vi "数组的更多使用3.vi"() -> ()   [LabVIEW 2025]
uses:
  87c27d12-5d39-4814-956f-28ff39b3eca0.vi
  7a71da50-a804-472e-9fb4-ea32467be636.vi
  161af4c8-741e-4c3b-a09d-9f8106a9c38e.vi
  <vilib>/Array/Sort 2D Array - Pop Stack.vi
  <vilib>/Array/Sort 2D Array - Push Stack.vi
  7a71da50-a804-472e-9fb4-ea32467be636.vi/269d4b3b-47f5-49e3-8884-44851e4dd9d5.vi
  7a71da50-a804-472e-9fb4-ea32467be636.vi/6d99389c-673d-4efb-bf33-19b32bcf4cf8.vi
panel:
  out "数组 4":cluster{"数值":dbl, "字符串":string}[](array[cluster])
  in  "数组 3":T1(array[cluster])
  out "簇 3":cluster{"数值":dbl, "字符串":string}
  out "数值 2":dbl
  out "字符串":string
  out "数值":dbl
  out "布尔":bool
  in  "簇 2":T2
  in  "数组":T1(array[cluster])
  out "簇":T2
  out "转置的数组":dbl[][](array[numeric])
  out "shuffled array 2":dbl[][](array[numeric]) caption="重排后数组"
  out "sorted 2D array":dbl[][](array[numeric]) caption="排序后的二维数组"
  out "index out of range?":bool caption="索引超出范围？"
  in  "dimension to index (column)":enum16{"column", "row"}(ring) caption="要索引的维度（列）"
  in  "index":i32 caption="索引"
  in  "二维数组":dbl[][](array[numeric])
  out "y值":dbl
  in  "分数索引":dbl
  out "降采样的数组 2":dbl[](array[numeric])
  out "降采样的数组 1":dbl[](array[numeric])
  in  "数组 2":dbl[](array[numeric])
  out "交织的数组":dbl[](array[numeric])
  in  "第n个元素":dbl
  out "数组（最后n个元素置于前端）":dbl[](array[numeric])
  out "shuffled array":dbl[](array[numeric]) caption="重排一维数组"
  out "1维数组排序":dbl[](array[numeric])
  in  "数组 1":dbl[](array[numeric])
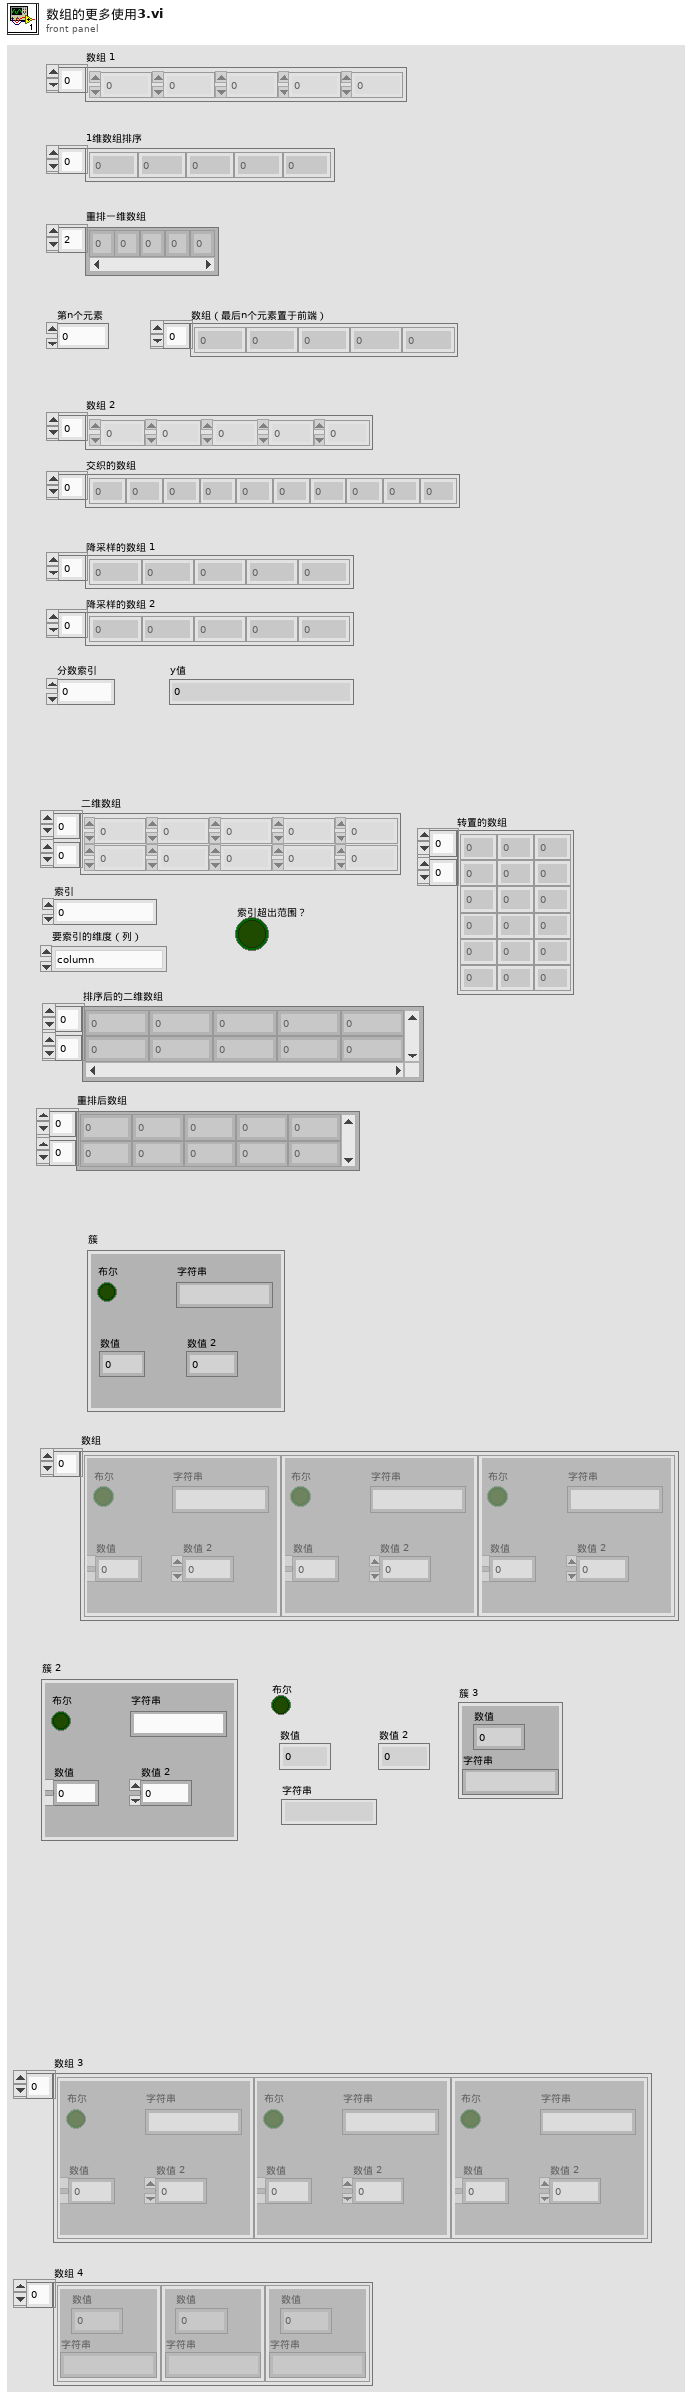
[diagram p1: front panel]
types:
  T1 = cluster{"布尔":bool, "数值":dbl, "字符串":string, "数值 2":dbl}[]
  T2 = cluster{"布尔":bool, "数值":dbl, "字符串":string, "数值 2":dbl}
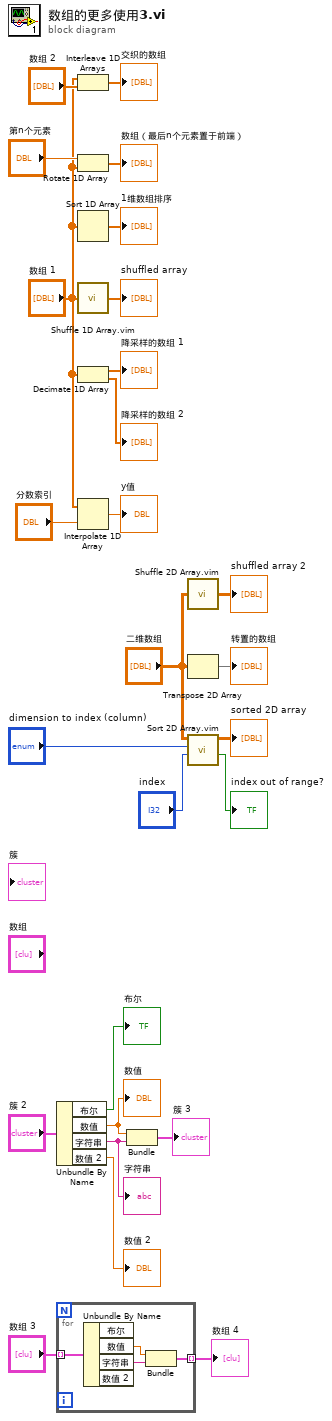
[diagram p0: block diagram]
diagram:
  n1 = Unbundle By Name("簇 2") -> ("布尔"=→"布尔":bool, "数值"=w5:dbl, "字符串"=w4:string, "数值 2"=→"数值 2":dbl)
  "数值" <- w5
  "字符串" <- w4
  n2 = for {
    tunnel: "数组 3" -> [w30] mode=indexing
    tunnel: [w27] -> w1 mode=indexing
    n3 = Unbundle By Name(w30) -> ("数值"=w29:dbl, "字符串"=w28:string)  [unwired: 2 out]
    n4 = Bundle("数值"=w29, "字符串"=w28) -> (w27:cluster{"数值":dbl, "字符串":string})  [unwired: 1 in]
  }
  "数组 4" <- w1
  n5 = Interleave 1D Arrays("数组 1", "数组 2") -> (→"交织的数组":dbl[])
  n6 = Rotate 1D Array(1:"数组 1", 2:"第n个元素") -> (0:→"数组（最后n个元素置于前端）":dbl[])
  n7 = Sort 1D Array(array="数组 1") -> (sorted array=→"1维数组排序":dbl[])
  n8 = call "Shuffle 1D Array.vim"("array"="数组 1") -> ("shuffled array"=→"shuffled array":dbl[])  [unwired: 4 in]
  n9 = Decimate 1D Array("数组 1") -> (→"降采样的数组 1":dbl[], →"降采样的数组 2":dbl[])
  n10 = Interpolate 1D Array(1:"分数索引", 2:"数组 1") -> (0:→"y值":dbl)
  n11 = Bundle("数值"=w5, "字符串"=w4) -> (→"簇 3":cluster{"数值":dbl, "字符串":string})  [unwired: 1 in]
  n12 = call "Shuffle 2D Array.vim"("array"="二维数组") -> ("shuffled array"=→"shuffled array 2":dbl[][])  [unwired: 4 in]
  n13 = Transpose 2D Array(2D array="二维数组") -> (transposed array=→"转置的数组":dbl[][])
  n14 = call "Sort 2D Array.vim"("index"="index", "dimension to index (column)"="dimension to index (column)", "2D array"="二维数组") -> ("index out of range?"=→"index out of range?":bool, "sorted 2D array"=→"sorted 2D array":dbl[][])  [unwired: 7 in]
